vi "Facade.vi"(0 "Data In":T5, 2 "Display State In":T3, 3 "Container State":T4) -> (6 "Data Out":T5, 7 "Display State Out":T3, 8 "Action":T2)   [LabVIEW 2017, in "Test Signal Configuration.xctl"]
uses:
  <vilib>/addons/_XControls/Function Generator Configuration/Test Signal Configuration.xctl
  <vilib>/addons/_XControls/Function Generator Configuration/Controls/Data.ctl
  <vilib>/addons/_NISVFA/_Generation/Signal Generation/SV Signal/SV Signal.lvclass
  <vilib>/_xctls/Container State.ctl
  <vilib>/addons/_XControls/Function Generator Configuration/Controls/State.ctl
  <vilib>/_xctls/Action.ctl
  <vilib>/addons/_XControls/Function Generator Configuration/Controls/signal type.ctl
  <vilib>/addons/_XControls/Function Generator Configuration/Controls/references.ctl
  <vilib>/_xctls/XControlSupport.lvlib
panel:
  in  "signal type":T1=enum."Tone"
  in  "Offset":dbl(slide) min=-2.0 max=2.0 step=0.1 scale=-2.0..2.0 scale format="%#_4g"
  in  "Amplitude":dbl(slide)=1.0 min=0.0 max=2.0 step=0.1 scale=0.0..2.0 scale format="%#_4g"
  out "signal type tab":T6(tab)=enum."Tone"
  in  "Frequency ( f )":dbl(slide)=997.0 min=20.0 max=20000.0 step=10.0 scale=20.0..20000.0 scale format="%#_3p"
  in  "multitone info":T7(array[cluster])=[{"frequency"=1000.0, "amplitude"=1.0, "phase"=100.0}, {"frequency"=1000.0, "amplitude"=1.0, "phase"=100.0}, {"frequency"=1000.0, "amplitude"=1.0, "phase"=100.0}, {"frequency"=1000.0, "amplitude"=1.0, "phase"=100.0}] {"phase" format="%#.1f°"; "amplitude" format="%#_5g"; "frequency" min=20.0 max=20000.0 format="%#_5p Hz"}
  in  "Steps":i32=100 min=1
  in  "Cycles | Time":dbl=1.0 min=0.5 max=1000.0 step=0.5
  in  "Spacing":u16(ring)=1 items=["Linear", "Logarithmic "]
  in  "Stop":dbl=8000.0 min=20.0 max=20000.0 format="%#_g Hz"
  in  "Start ( f 0 )":dbl=100.0 min=20.0 max=20000.0 format="%#_g Hz"
  in  "Measurement Time":dbl=1.0 min=0.0 max=10.0 step=0.001 format="%#_g s"
  in  "Duration":dbl=1.0 min=0.02 max=10.0 step=0.001 format="%#_g s"
  in  "Profile":u16(ring)=1 items=["Linear", "Logarithmic"]
  in  "cs_Stop":dbl=8000.0 caption="Stop" min=20.0 max=20000.0 format="%#_g Hz"
  in  "cs_Start (f0)":dbl=100.0 caption="Start ( f 0 )" min=20.0 max=20000.0 format="%#_g Hz"
  in  "Seed":i32=-1
  in  "Density Function":enum16{"White", "Pink"}(ring)
  # "To enable this configuration, \nselect a dynamic signal type."
  # "f i"
  # "a i"
  # "f i"
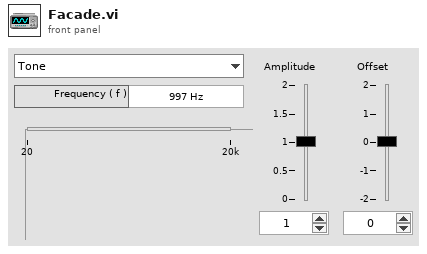
[diagram p1: front panel]
types:
  T1 = typedef "Test Signal Configuration.xctl/signal type.ctl" = enum32{"None", "Tone", "Multitone", "Discrete Sweep", "Continuous Sweep", "Noise"}
  T2 = typedef "XControlSupport.lvlib/Action.ctl" = cluster{"Data Changed?":bool, "State Changed?":bool, "Action Name":string}
  T3 = typedef "Test Signal Configuration.xctl/State.ctl" = cluster{"Attributes":variant}
  T4 = typedef "XControlSupport.lvlib/Container State.ctl" = cluster{"Indicator?":bool, "Run Mode?":bool, " Refnum":refnum<vi>}
  T5 = typedef "Test Signal Configuration.xctl/Data.ctl" = refnum<class "SV Signal.lvclass">
  T6 = enum32{"None", "Tone", "Multitone", "Discrete Sweep", "Continuous Sweep", "Noise"}
  T7 = cluster{"frequency":dbl, "amplitude":dbl, "phase":dbl}[]
  T8 = typedef "Test Signal Configuration.xctl/references.ctl" = cluster{"signal":cluster{"signal type":refnum<vi>, "signal type tab":refnum<vi>, "Amplitude":refnum<vi>, "Offset":refnum<vi>}, "function":cluster{"Frequency (f)":refnum<vi>}, "continuous sweep":cluster{"cs_Start (f0)":refnum<vi>, "cs_Stop":refnum<vi>, "Duration":refnum<vi>, "Profile":refnum<vi>}, "discrete sweep":cluster{"Start (f0)":refnum<vi>, "Stop":refnum<vi>, "Steps":refnum<vi>, "Spacing":refnum<vi>, "Cycles | Time":refnum<vi>, "Measurement Time":refnum<vi>}, "multitone":cluster{"multitone info":refnum<vi>, "multitone.frequency":refnum<vi>}, "noise":cluster{"Density Function":refnum<vi>, "Seed":refnum<vi>}}
  T9 = cluster{"signal type":refnum<vi>, "signal type tab":refnum<vi>, "Amplitude":refnum<vi>, "Offset":refnum<vi>}
  T10 = cluster{"Start (f0)":refnum<vi>, "Stop":refnum<vi>, "Steps":refnum<vi>, "Spacing":refnum<vi>, "Cycles | Time":refnum<vi>, "Measurement Time":refnum<vi>}
  T11 = cluster{"cs_Start (f0)":refnum<vi>, "cs_Stop":refnum<vi>, "Duration":refnum<vi>, "Profile":refnum<vi>}
  T12 = cluster{"multitone info":refnum<vi>, "multitone.frequency":refnum<vi>}
  T13 = cluster{"Density Function":refnum<vi>, "Seed":refnum<vi>}
  T14 = cluster{"Data Changed?":refnum<user-event>, "State Changed?":refnum<user-event>}
  T15 = cluster{"Signal":cluster{"Sample Rate":cluster{"name":string, "default":dbl}, "Signal Type":cluster{"name":string, "signal type":T1}, "Amplitude":cluster{"name":string, "default":dbl}, "Offset":cluster{"name":string, "default":dbl}}, "Function":cluster{"Info":cluster{"name":string, "default":variant}, "Type":cluster{"name":string, "default":u16}, "Frequency":cluster{"name":string, "default":dbl}, "Phase":cluster{"name":string, "default":dbl}}, "Continuous Sweep":cluster{"Info":cluster{"name":string, "default":variant}, "Start":cluster{"name":string, "default":dbl}, "Stop":cluster{"name":string, "default":dbl}, "Duration":cluster{"name":string, "default":dbl}, "Profile":cluster{"name":string, "default":enum16{"Linear", "Logarithmic"}}}, "Discrete Sweep":cluster{"Info":cluster{"name":string, "default":variant}, "Start":cluster{"name":string, "default":dbl}, "Stop":cluster{"name":string, "default":dbl}, "Cycles":cluster{"name":string, "default":dbl}, "Time":cluster{"name":string, "default":dbl}, "Spacing":cluster{"name":string, "default":enum16{"Linear", "Logarithmic"}}, "Steps":cluster{"name":string, "default":i32}}, "Multitone":cluster{"Info":cluster{"name":string, "multitone info":cluster{"frequency":dbl, "amplitude":dbl, "phase":dbl}[]}}, "Noise":cluster{"Info":cluster{"name":string, "default":variant}, "Type":cluster{"name":string, "default":u16}, "Amplitude PDF":cluster{"name":string, "default":enum16{"Gaussian", "Rectangular", "Triangular"}}, "Level":cluster{"name":string, "default":dbl}, "Seed":cluster{"name":string, "default":i32}}, "Configuration":cluster{"Min Frequency":cluster{"name":string, "default":dbl}, "Max Frequency":cluster{"name":string, "default":dbl}, "Max Amplitude":cluster{"name":string, "default":dbl}}}
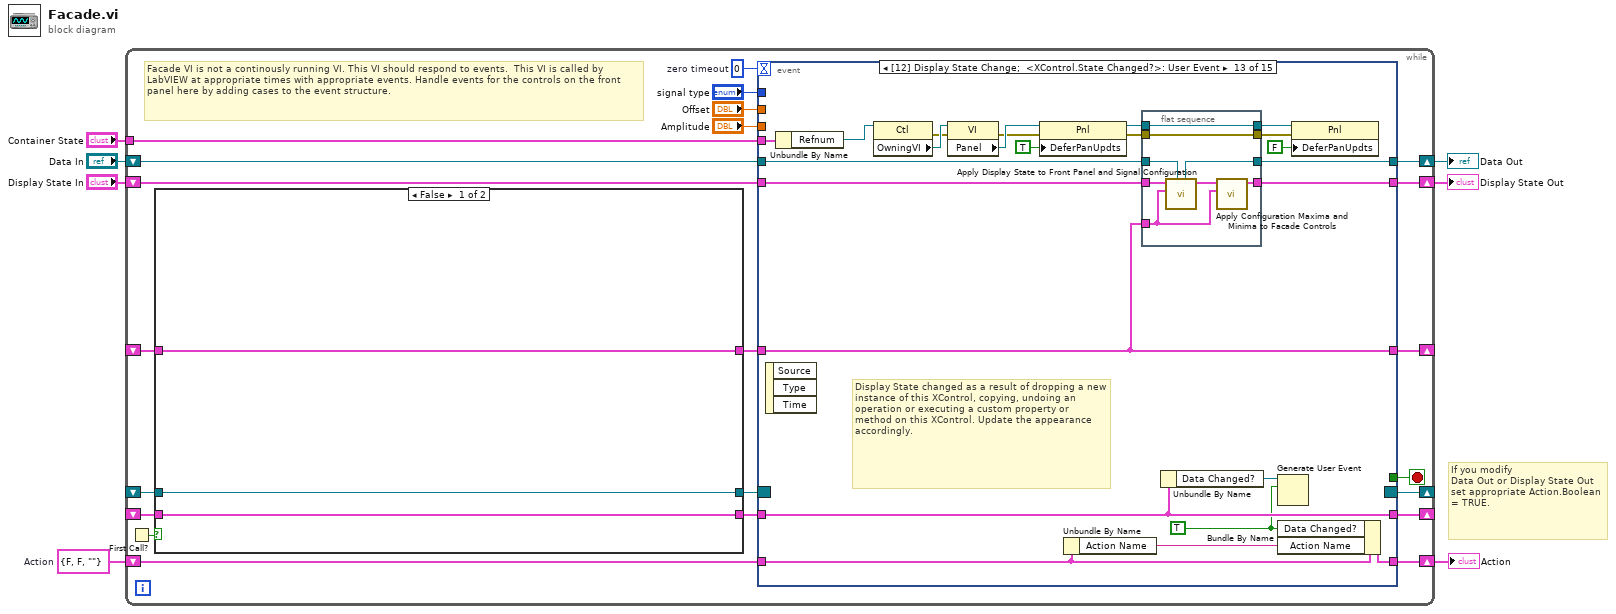
[diagram p0: block diagram]
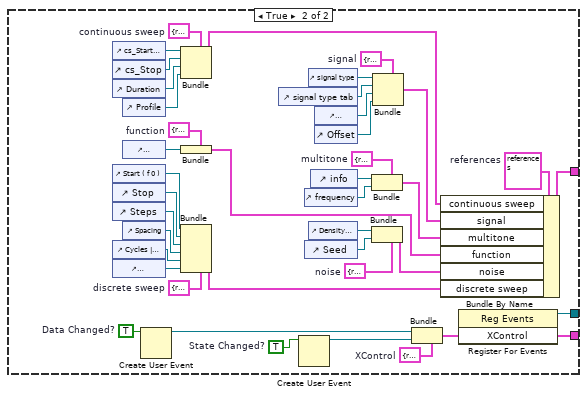
[diagram p2: hidden frame]
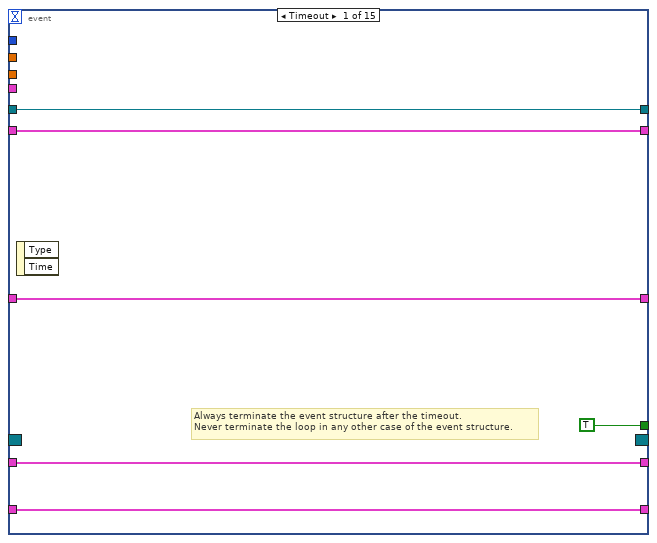
[diagram p3: hidden frame]
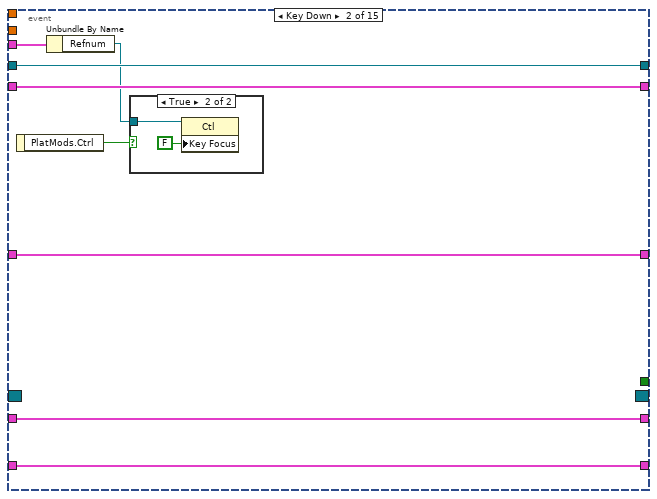
[diagram p4: hidden frame]
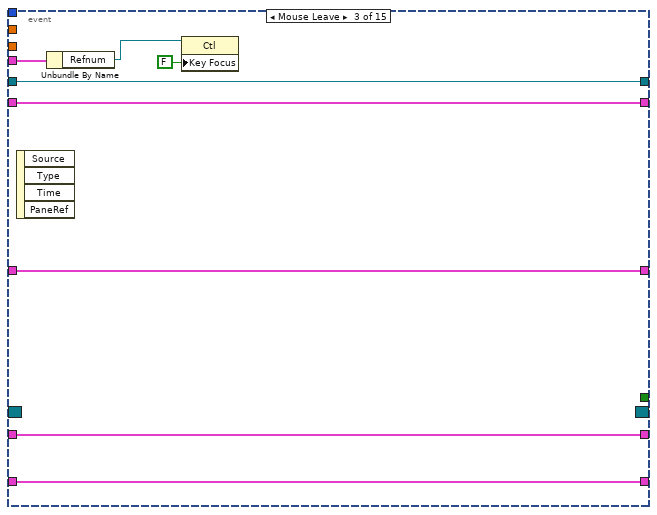
[diagram p6: hidden frame]
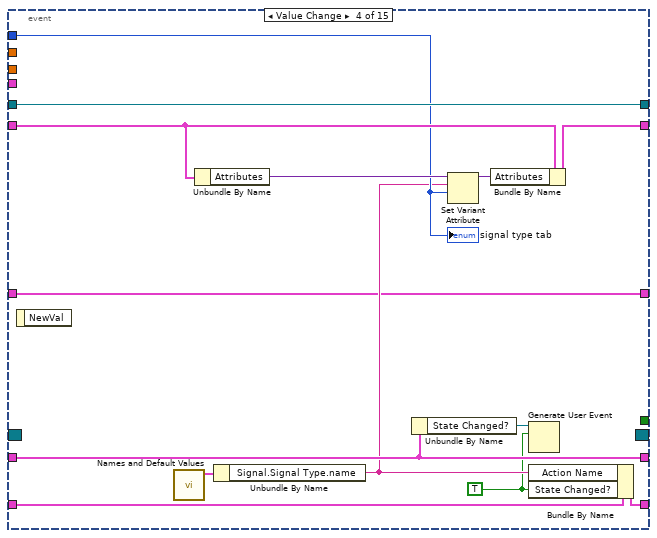
[diagram p7: hidden frame]
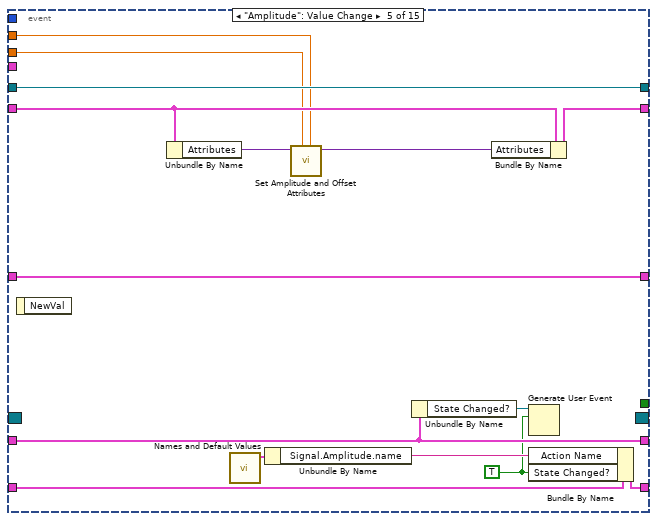
[diagram p8: hidden frame]
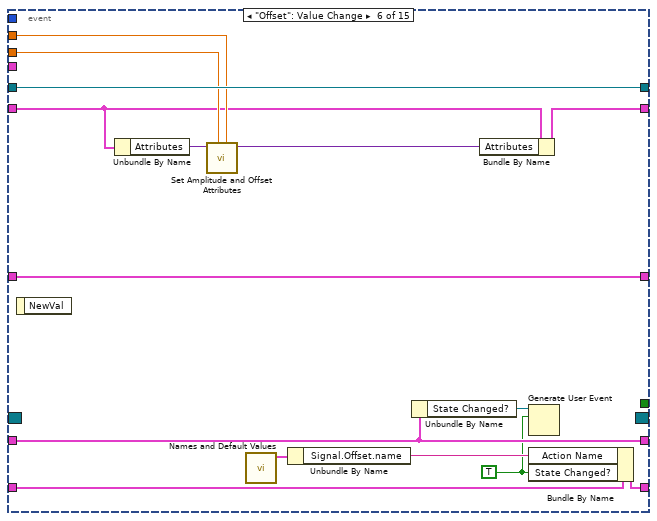
[diagram p9: hidden frame]
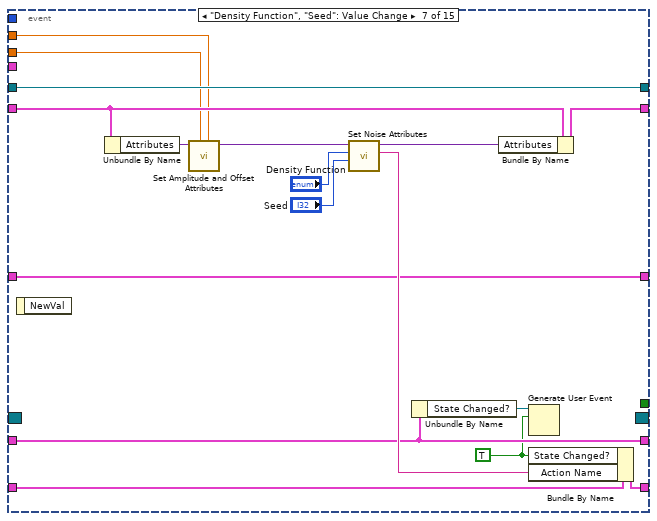
[diagram p10: hidden frame]
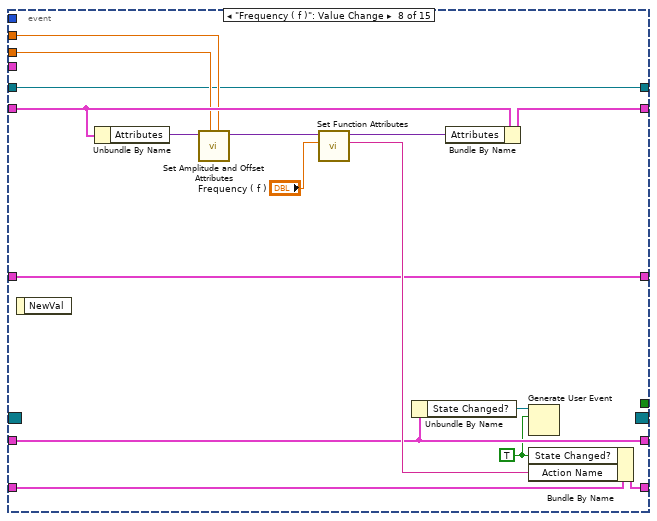
[diagram p11: hidden frame]
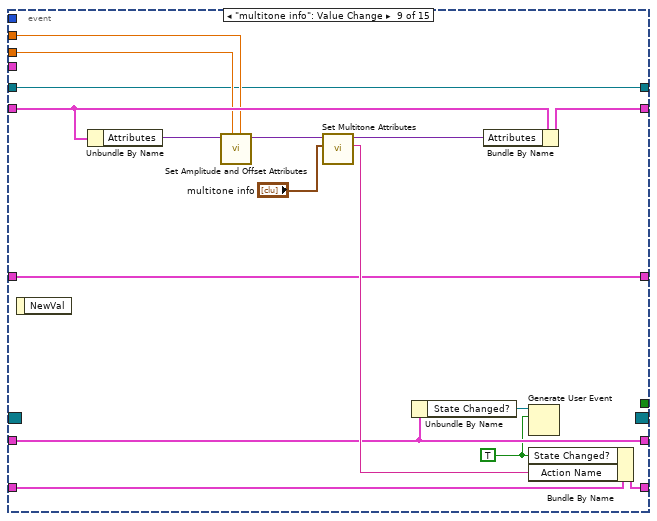
[diagram p12: hidden frame]
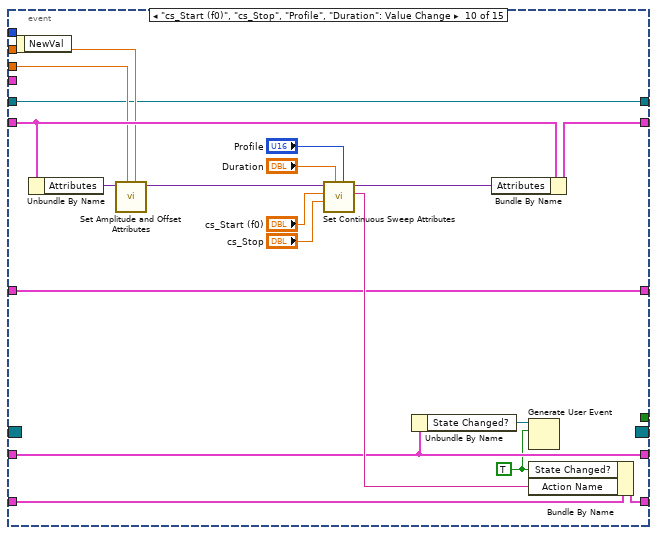
[diagram p13: hidden frame]
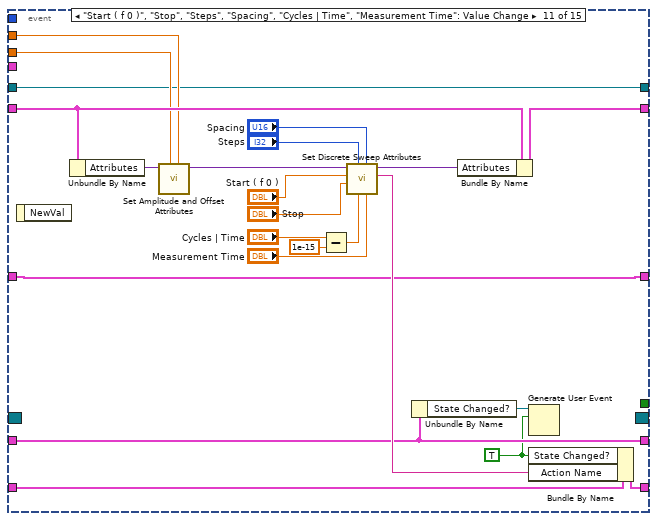
[diagram p14: hidden frame]
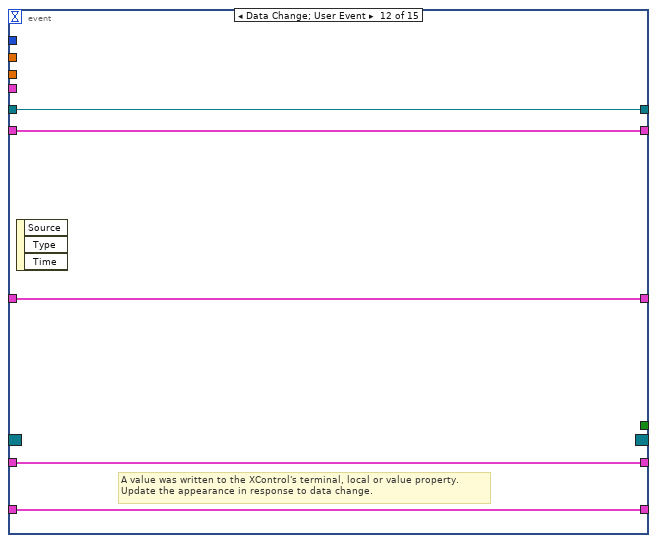
[diagram p15: hidden frame]
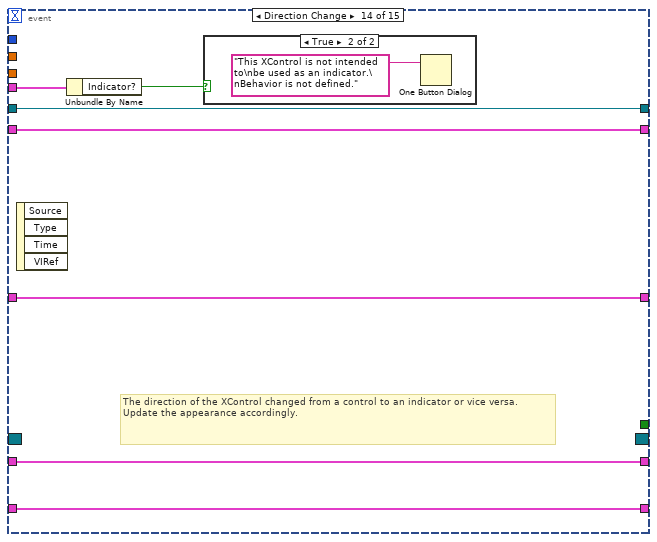
[diagram p16: hidden frame]
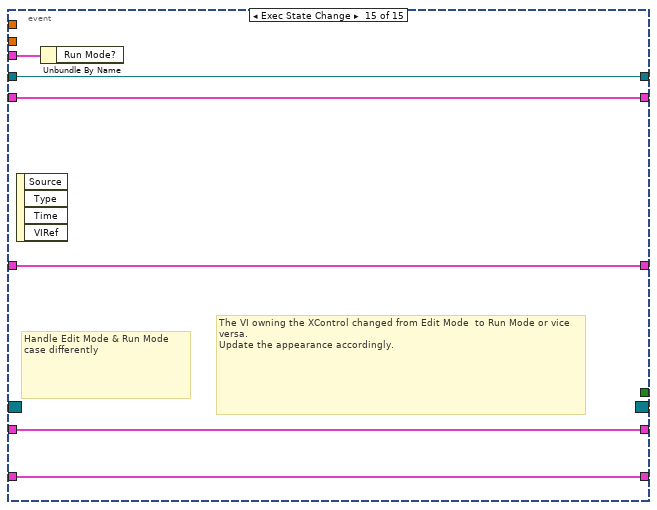
[diagram p18: hidden frame]
diagram:
  w1 = T2 {"Data Changed?"=FALSE, "State Changed?"=FALSE, "Action Name"=""}  # Action
  # "If you modify \nData Out or Display State Out set appropriate Action.Boolean = TRUE."
  n1 = while {
    shift-right: [w28] -> w4
    shift-left: "Display State In" -> [w29]
    tunnel: "Container State" -> [w25]
    shift-right: [w18] -> w7
    shift-left: "Data In" -> [w24]
    shift-right: [w22] -> w2
    shift-left: w1 -> [w23]
    shift-right: [w16] -> _
    shift-left: _ -> [w14]
    shift-right: [w12] -> _
    shift-left: _ -> [w11]
    shift-right: [w9] -> _
    shift-left: _ -> [w8]
    stop <- w27 stop-if-true
    w26 = 0  # zero timeout
    # "Facade VI is not a continously running VI. This VI should respond to events.  This VI is called by LabVIEW at appropriate times with appropriate events. Handle events for the controls on the front panel here by adding cases to the event structure."
    n2 = First Call?() -> (First Call?: T/F=w17:bool)
    n3 = case shown="False" w17 {
      tunnel: [w32 w70] -> w15
      tunnel: w14 -> [w32 _]
      tunnel: [w31 w66] -> w13
      tunnel: w11 -> [w31 _]
      tunnel: [w30 w34] -> w10
      tunnel: w8 -> [w30 _]
      frame False {
      }
      frame True {
        w60 = T8 {"signal"={"signal type"=refnum, "signal type tab"=refnum, "Amplitude"=refnum, "Offset"=refnum}, "function"={"Frequency (f)"=refnum}, "continuous sweep"={"cs_Start (f0)"=refnum, "cs_Stop"=refnum, "Duration"=refnum, "Profile"=refnum}, "discrete sweep"={"Start (f0)"=refnum, "Stop"=refnum, "Steps"=refnum, "Spacing"=refnum, "Cycles | Time"=refnum, "Measurement Time"=refnum}, "multitone"={"multitone info"=refnum, "multitone.frequency"=refnum}, "noise"={"Density Function"=refnum, "Seed"=refnum}}  # references
        w58 = T9 {"signal type"=refnum, "signal type tab"=refnum, "Amplitude"=refnum, "Offset"=refnum}  # signal
        w57 = T10 {"Start (f0)"=refnum, "Stop"=refnum, "Steps"=refnum, "Spacing"=refnum, "Cycles | Time"=refnum, "Measurement Time"=refnum}  # discrete sweep
        w50 = T11 {"cs_Start (f0)"=refnum, "cs_Stop"=refnum, "Duration"=refnum, "Profile"=refnum}  # continuous sweep
        w46 = T12 {"multitone info"=refnum, "multitone.frequency"=refnum}  # multitone
        w42 = cluster{"Frequency (f)":refnum<vi>} {"Frequency (f)"=refnum}  # function
        w40 = T13 {"Density Function"=refnum, "Seed"=refnum}  # noise
        w67 = T14 {"Data Changed?"=refnum, "State Changed?"=refnum}  # XControl
        w71 = TRUE  # State Changed?
        w72 = TRUE  # Data Changed?
        n4 = control-ref of="cs_Start (f0)"() -> (w37:refnum<vi>)
        n5 = control-ref of="cs_Stop"() -> (w47:refnum<vi>)
        n6 = control-ref of="Duration"() -> (w48:refnum<vi>)
        n7 = control-ref of="Start ( f 0 )"() -> (w51:refnum<vi>)
        n8 = control-ref of="Stop"() -> (w52:refnum<vi>)
        n9 = control-ref of="Steps"() -> (w53:refnum<vi>)
        n10 = control-ref of="Cycles | Time"() -> (w55:refnum<vi>)
        n11 = control-ref of="Measurement Time"() -> (w56:refnum<vi>)
        n12 = control-ref of="Profile"() -> (w49:refnum<vi>)
        n13 = control-ref of="Frequency ( f )"() -> (w41:refnum<vi>)
        n14 = control-ref of="Spacing"() -> (w54:refnum<vi>)
        n15 = Create User Event(user event datatype=w72) -> (user event=w69:refnum<user-event>)  [unwired: 1 in, 1 out]
        n16 = Bundle(cluster=w50, "cs_Start (f0)"=w37, "cs_Stop"=w47, "Duration"=w48, "Profile"=w49) -> (w63:T11)
        n17 = Bundle(cluster=w42, "Frequency (f)"=w41) -> (w65:cluster{"Frequency (f)":refnum<vi>})
        n18 = Bundle(cluster=w57, "Start (f0)"=w51, "Stop"=w52, "Steps"=w53, "Spacing"=w54, "Cycles | Time"=w55, "Measurement Time"=w56) -> (w61:T10)
        n19 = control-ref of="signal type tab"() -> (w64:refnum<vi>)
        n20 = Create User Event(user event datatype=w71) -> (user event=w68:refnum<user-event>)  [unwired: 1 in, 1 out]
        n21 = control-ref of="frequency"() -> (w45:refnum<vi>)
        n22 = control-ref of="Seed"() -> (w39:refnum<vi>)
        n23 = control-ref of="signal type"() -> (w43:refnum<vi>)
        n24 = control-ref of="Density Function"() -> (w38:refnum<vi>)
        n25 = control-ref of="info"() -> (w44:refnum<vi>)
        n26 = control-ref of="Amplitude"() -> (w35:refnum<vi>)
        n27 = control-ref of="Offset"() -> (w36:refnum<vi>)
        n28 = Bundle(cluster=w46, "multitone info"=w44, "multitone.frequency"=w45) -> (w59:T12)
        n29 = Bundle(cluster=w40, "Density Function"=w38, "Seed"=w39) -> (w62:T13)
        n30 = Bundle(cluster=w58, "signal type"=w43, "signal type tab"=w64, "Amplitude"=w35, "Offset"=w36) -> (w33:T9)
        n31 = Bundle(cluster=w67, "Data Changed?"=w69, "State Changed?"=w68) -> (w66:T14)
        n32 = Bundle By Name(cluster=w60, "continuous sweep"=w63, "signal"=w33, "multitone"=w59, "function"=w65, "noise"=w62, "discrete sweep"=w61) -> (w34:T8)
        n33 = register-events(w66) -> (reference out=w70:refnum<event-registration>)  [unwired: 2 in, 1 out]
      }
    }
    n34 = event shown="[12] Display State Change;  <XControl.State Changed?>: User Event" {
      selector: w15 -> [_ _ _ _ _ _ _ _ _ _ _ _ _ _ _]
      dyn-events: [_ _ _ _ _ _ _ _ _ _ _ _ _ _ _] -> w16
      timeout: w26 -> [_ _ _ _ _ _ _ _ _ _ _ _ _ _ _]
      tunnel: w29 -> [w76 w86 w96 w106 w122 w131 w156 w172 w186 w206 w230 w236 w256 w273 w280]
      tunnel: [w76 w86 w96 w105 w121 w137 w155 w171 w188 w205 w229 w236 w259 w273 w280] -> w28
      tunnel: [TRUE _ _ _ _ _ _ _ _ _ _ _ _ _ _] -> w27
      tunnel: w25 -> [_ w81 w91 _ _ _ _ _ _ _ _ _ w248 w274 w281]
      tunnel: w24 -> [w75 w85 w95 w110 w125 w140 w157 w167 w178 w200 w217 w234 w258 w272 w279]
      tunnel: [w75 w85 w95 w110 w125 w140 w157 w167 w178 w200 w217 w234 w257 w272 w279] -> w18
      tunnel: [w77 w84 w94 w103 w123 w138 w153 w162 w184 w207 w222 w235 w255 w271 w278] -> w22
      tunnel: w23 -> [w77 w84 w94 w107 w124 w139 w154 w173 w185 w208 w231 w235 w254 w271 w278]
      tunnel: "Amplitude" -> [_ _ _ _ w118 w133 w151 w169 w181 w203 w228 _ _ _ _]
      tunnel: "Offset" -> [_ _ _ _ w117 w134 w150 w168 w180 w202 w221 _ _ _ _]
      tunnel: "signal type" -> [_ _ _ w102 _ _ _ _ _ _ _ _ _ _ _]
      tunnel: w10 -> [w73 w82 w92 w97 w111 w126 w141 w158 w174 w190 w209 w232 w249 w268 w276]
      tunnel: w13 -> [w74 w83 w93 w100 w114 w128 w143 w160 w176 w192 w211 w233 w251 w269 w277]
      tunnel: [w74 w83 w93 w100 w114 w128 w143 w160 w176 w192 w211 w233 w251 w269 w277] -> w12
      tunnel: [w73 w82 w92 w97 w111 w126 w141 w158 w174 w190 w209 w232 w249 w268 w276] -> w9
      event Timeout {
        # "Always terminate the event structure after the timeout. \nNever terminate the loop in any other case of the event structure."
        n35 = event-data() -> ()  [unwired: 1 in, 2 out]
      }
      event Key Down {
        n36 = event-data() -> ("PlatMods.Ctrl"=w79:bool)  [unwired: 1 in]
        n37 = Unbundle By Name(w81) -> ("Refnum"=w80:refnum<vi>)
        n38 = case shown="True" w79 {
          tunnel: w80 -> [_ w88]
          frame False {
          }
          frame True {
            n39 = property class="Ctl"(reference=w88, "Key Focus"=FALSE) -> ()  [unwired: 1 in, 2 out]
          }
        }
      }
      event Mouse Leave {
        n40 = event-data() -> ()  [unwired: 1 in, 4 out]
        n41 = Unbundle By Name(w91) -> ("Refnum"=w90:refnum<vi>)
        n42 = property class="Ctl"(reference=w90, "Key Focus"=FALSE) -> ()  [unwired: 1 in, 2 out]
      }
      event Value Change {
        w98 = TRUE ("State Changed?")
        n43 = event-data() -> ()  [unwired: 1 in, 1 out]
        n44 = call <vilib>:"Names and Default Values.vi"() -> ("Names and Default Values"=w104:T15)  [unwired: 11 in]
        n45 = Unbundle By Name(w106) -> ("Attributes"=w109:variant)
        n46 = Unbundle By Name(w104) -> ("Signal.Signal Type.name"=w99:string)
        n47 = Unbundle By Name(w100) -> ("State Changed?"=w101:refnum<user-event>)
        n48 = Set Variant Attribute(Variant=w109, name=w99, value=w102) -> (Variant out=w108:variant)  [unwired: 1 in, 2 out]
        n49 = Bundle By Name(cluster=w106, "Attributes"=w108) -> (w105:T3)
        n50 = Generate User Event(user event=w101, event data cluster=w98) -> ()  [unwired: 2 in, 2 out]
        n51 = Bundle By Name(cluster=w107, "Action Name"=w99, "State Changed?"=w98) -> (w103:T2)
        "signal type tab" <- w102
      }
      event "Amplitude": Value Change {
        w112 = TRUE ("State Changed?")
        n52 = event-data() -> ()  [unwired: 1 in, 1 out]
        n53 = Unbundle By Name(w122) -> ("Attributes"=w120:variant)
        n54 = call <vilib>:"Names and Default Values.vi"() -> ("Names and Default Values"=w116:T15)  [unwired: 11 in]
        n55 = Unbundle By Name(w116) -> ("Signal.Amplitude.name"=w113:string)
        n56 = call <vilib>:"Set Amplitude and Offset Attributes.vi"("Offset"=w117, "Amplitude"=w118, "Display State Attributes in"=w120) -> ("Display State Attributes out"=w119:variant)  [unwired: 5 in, 1 out]
        n57 = Unbundle By Name(w114) -> ("State Changed?"=w115:refnum<user-event>)
        n58 = Bundle By Name(cluster=w122, "Attributes"=w119) -> (w121:T3)
        n59 = Generate User Event(user event=w115, event data cluster=w112) -> ()  [unwired: 2 in, 2 out]
        n60 = Bundle By Name(cluster=w124, "Action Name"=w113, "State Changed?"=w112) -> (w123:T2)
      }
      event "Offset": Value Change {
        w127 = TRUE ("State Changed?")
        n61 = event-data() -> ()  [unwired: 1 in, 1 out]
        n62 = Unbundle By Name(w131) -> ("Attributes"=w136:variant)
        n63 = call <vilib>:"Set Amplitude and Offset Attributes.vi"("Offset"=w134, "Amplitude"=w133, "Display State Attributes in"=w136) -> ("Display State Attributes out"=w135:variant)  [unwired: 5 in, 1 out]
        n64 = call <vilib>:"Names and Default Values.vi"() -> ("Names and Default Values"=w132:T15)  [unwired: 11 in]
        n65 = Unbundle By Name(w132) -> ("Signal.Offset.name"=w130:string)
        n66 = Unbundle By Name(w128) -> ("State Changed?"=w129:refnum<user-event>)
        n67 = Bundle By Name(cluster=w131, "Attributes"=w135) -> (w137:T3)
        n68 = Generate User Event(user event=w129, event data cluster=w127) -> ()  [unwired: 2 in, 2 out]
        n69 = Bundle By Name(cluster=w139, "Action Name"=w130, "State Changed?"=w127) -> (w138:T2)
      }
      event "Density Function", "Seed": Value Change {
        w142 = TRUE ("State Changed?")
        n70 = event-data() -> ()  [unwired: 1 in, 1 out]
        n71 = Unbundle By Name(w156) -> ("Attributes"=w152:variant)
        n72 = call <vilib>:"Set Amplitude and Offset Attributes.vi"("Offset"=w150, "Amplitude"=w151, "Display State Attributes in"=w152) -> ("Display State Attributes out"=w146:variant)  [unwired: 5 in, 1 out]
        n73 = call <vilib>:"Set Noise Attributes.vi"("Seed"="Seed", "Density Function"="Density Function", "Display State Attributes in"=w146) -> ("name"=w149:string, "Display State Attributes out"=w145:variant)  [unwired: 7 in]
        n74 = Unbundle By Name(w143) -> ("State Changed?"=w144:refnum<user-event>)
        n75 = Bundle By Name(cluster=w156, "Attributes"=w145) -> (w155:T3)
        n76 = Generate User Event(user event=w144, event data cluster=w142) -> ()  [unwired: 2 in, 2 out]
        n77 = Bundle By Name(cluster=w154, "State Changed?"=w142, "Action Name"=w149) -> (w153:T2)
      }
      event "Frequency ( f )": Value Change {
        w159 = TRUE ("State Changed?")
        n78 = event-data() -> ()  [unwired: 1 in, 1 out]
        n79 = Unbundle By Name(w172) -> ("Attributes"=w170:variant)
        n80 = call <vilib>:"Set Amplitude and Offset Attributes.vi"("Offset"=w168, "Amplitude"=w169, "Display State Attributes in"=w170) -> ("Display State Attributes out"=w165:variant)  [unwired: 5 in, 1 out]
        n81 = call <vilib>:"Set Function Attributes.vi"("Frequency (f)"="Frequency ( f )", "Display State Attributes in"=w165) -> ("name"=w163:string, "Display State Attributes out"=w164:variant)  [unwired: 8 in]
        n82 = Unbundle By Name(w160) -> ("State Changed?"=w161:refnum<user-event>)
        n83 = Bundle By Name(cluster=w172, "Attributes"=w164) -> (w171:T3)
        n84 = Generate User Event(user event=w161, event data cluster=w159) -> ()  [unwired: 2 in, 2 out]
        n85 = Bundle By Name(cluster=w173, "State Changed?"=w159, "Action Name"=w163) -> (w162:T2)
      }
      event "multitone info": Value Change {
        w175 = TRUE ("State Changed?")
        n86 = event-data() -> ()  [unwired: 1 in, 1 out]
        n87 = Unbundle By Name(w186) -> ("Attributes"=w183:variant)
        n88 = call <vilib>:"Set Amplitude and Offset Attributes.vi"("Offset"=w180, "Amplitude"=w181, "Display State Attributes in"=w183) -> ("Display State Attributes out"=w182:variant)  [unwired: 5 in, 1 out]
        n89 = call <vilib>:"Set Multitone Attributes.vi"("multitone info"="multitone info", "Display State Attributes in"=w182) -> ("name"=w179:string, "Display State Attributes out"=w189:variant)  [unwired: 8 in]
        n90 = Unbundle By Name(w176) -> ("State Changed?"=w177:refnum<user-event>)
        n91 = Bundle By Name(cluster=w186, "Attributes"=w189) -> (w188:T3)
        n92 = Generate User Event(user event=w177, event data cluster=w175) -> ()  [unwired: 2 in, 2 out]
        n93 = Bundle By Name(cluster=w185, "State Changed?"=w175, "Action Name"=w179) -> (w184:T2)
      }
      event "cs_Start (f0)", "cs_Stop", "Profile", "Duration": Value Change {
        w191 = TRUE ("State Changed?")
        n94 = event-data() -> ()  [unwired: 1 in, 1 out]
        n95 = Unbundle By Name(w206) -> ("Attributes"=w204:variant)
        n96 = call <vilib>:"Set Amplitude and Offset Attributes.vi"("Offset"=w202, "Amplitude"=w203, "Display State Attributes in"=w204) -> ("Display State Attributes out"=w197:variant)  [unwired: 5 in, 1 out]
        n97 = call <vilib>:"Set Continuous Sweep Attributes.vi"("Profile"="Profile", "Duration"="Duration", "stop"="cs_Stop", "start"="cs_Start (f0)", "Display State Attributes in"=w197) -> ("name"=w201:string, "Display State Attributes out"=w196:variant)  [unwired: 5 in]
        n98 = Unbundle By Name(w192) -> ("State Changed?"=w193:refnum<user-event>)
        n99 = Bundle By Name(cluster=w206, "Attributes"=w196) -> (w205:T3)
        n100 = Generate User Event(user event=w193, event data cluster=w191) -> ()  [unwired: 2 in, 2 out]
        n101 = Bundle By Name(cluster=w208, "State Changed?"=w191, "Action Name"=w201) -> (w207:T2)
      }
      event "Start ( f 0 )", "Stop", "Steps", "Spacing", "Cycles | Time", "Measurement Time": Value Change {
        w210 = TRUE ("State Changed?")
        n102 = event-data() -> ()  [unwired: 1 in, 1 out]
        n103 = Unbundle By Name(w230) -> ("Attributes"=w227:variant)
        n104 = call <vilib>:"Set Amplitude and Offset Attributes.vi"("Offset"=w221, "Amplitude"=w228, "Display State Attributes in"=w227) -> ("Display State Attributes out"=w215:variant)  [unwired: 5 in, 1 out]
        n105 = Subtract(x="Cycles | Time", y=1e-15) -> (x-y=w218:dbl)
        n106 = call <vilib>:"Set Discrete Sweep Attributes.vi"("Measurement Time"="Measurement Time", "Spacing"="Spacing", "Measurement Cycles"=w218, "Steps"="Steps", "stop"="Stop", "start"="Start ( f 0 )", "Display State Attributes in"=w215) -> ("name"=w223:string, "Display State Attributes out"=w216:variant)  [unwired: 3 in]
        n107 = Unbundle By Name(w211) -> ("State Changed?"=w212:refnum<user-event>)
        n108 = Bundle By Name(cluster=w230, "Attributes"=w216) -> (w229:T3)
        n109 = Generate User Event(user event=w212, event data cluster=w210) -> ()  [unwired: 2 in, 2 out]
        n110 = Bundle By Name(cluster=w231, "State Changed?"=w210, "Action Name"=w223) -> (w222:T2)
      }
      event Data Change; User Event {
        # "A value was written to the XControl's terminal, local or value property.\nUpdate the appearance in response to data change."
        n111 = event-data() -> ()  [unwired: 1 in, 3 out]
      }
      event Display State Change; User Event {
        w250 = TRUE ("State Changed?")
        # "Display State changed as a result of dropping a new instance of this XControl, copying, undoing an operation or executing a custom property or method on this XControl. Update the appearance accordingly."
        n112 = event-data() -> ()  [unwired: 1 in, 3 out]
        n113 = Unbundle By Name(w248) -> ("Refnum"=w241:refnum<vi>)
        n114 = property class="Ctl"(reference=w241) -> (error out=w244:errorcluster, "OwningVI"=w247:refnum<vi>)  [unwired: 1 in, 1 out]
        n115 = property class="VI"(reference=w247, error in=w244) -> (error out=w243:errorcluster, "Panel"=w246:refnum<vi>)  [unwired: 1 out]
        n116 = property class="Pnl"(reference=w246, error in=w243, "DeferPanUpdts"=TRUE ("Defer Panel Updates")) -> (reference out=w238:refnum<vi>, error out=w240:errorcluster)
        n117 = Unbundle By Name(w254) -> ("Action Name"=w253:string)
        n118 = flat-sequence {
          tunnel: [w267] -> w259
          tunnel: w258 -> [w266]
          tunnel: [w265] -> w257
          tunnel: w256 -> [w264]
          tunnel: w249 -> [w262]
          tunnel: w240 -> [w260]
          tunnel: [w261] -> w239
          tunnel: w238 -> [w261]
          tunnel: [w260] -> w237
          frame #0 {
            n119 = call <vilib>:"Apply Display State to Front Panel and Signal Configuration.vi"("Data In"=w266, "references"=w262, "Display State In"=w264) -> ("Display State Out"=w263:T3, "Data Out"=w265:T5)  [unwired: 7 in]
            n120 = call <vilib>:"Apply Configuration Maxima and Minima to Facade Controls.vi"("references"=w262, "Display State In"=w263) -> ("Display State Out"=w267:T3)  [unwired: 9 in]
          }
        }
        n121 = Unbundle By Name(w251) -> ("Data Changed?"=w252:refnum<user-event>)
        n122 = Generate User Event(user event=w252, event data cluster=w250) -> ()  [unwired: 2 in, 2 out]
        n123 = Bundle By Name(cluster=w254, "Data Changed?"=w250, "Action Name"=w253) -> (w255:T2)
        n124 = property class="Pnl"(reference=w239, error in=w237, "DeferPanUpdts"=FALSE ("Defer Panel Updates")) -> ()  [unwired: 2 out]
      }
      event Direction Change {
        # "The direction of the XControl changed from a control to an indicator or vice versa. Update the appearance accordingly."
        n125 = event-data() -> ()  [unwired: 1 in, 4 out]
        n126 = Unbundle By Name(w274) -> ("Indicator?"=w270:bool)
        n127 = case shown="True" w270 {
          frame False {
          }
          frame True {
            n128 = One Button Dialog(message="This XControl is not intended to\nbe used as an indicator.\nBehavior is not defined.") -> ()  [unwired: 1 in, 1 out]
          }
        }
      }
      event Exec State Change {
        # "The VI owning the XControl changed from Edit Mode  to Run Mode or vice versa.\nUpdate the appearance accordingly."
        # "Handle Edit Mode & Run Mode\ncase differently"
        n129 = event-data() -> ()  [unwired: 1 in, 4 out]
        n130 = Unbundle By Name(w281) -> ()  [unwired: 1 out]
      }
    }
  }
  "Display State Out" <- w4
  "Data Out" <- w7
  "Action" <- w2
